vi "Get Event Name.vi"(8 "error in (no error)":errorcluster {"code" format="%.0x"}, 9 "EventNameBufferSize":i32=256 caption="EventNameBufferSize (256)", 10 "EventIndex":i32=1 caption="EventIndex (1)" format="%.0g", 11 "instrument handle":refnum<k15>) -> (0 "error out":errorcluster {"code" format="%.0x"}, 2 "EventName":string, 3 "instrument handle out":refnum<k15>)   [LabVIEW 2009, in "Keysight XSAn.lvlib"]
doc: "This VI returns the physical repeated capability identifier that corresponds to the one-based index that the user specifies. If the value that the user passes for the EventIndex parameter is less than one or greater than the value of the Event Count property, the VI returns an empty string in the EventName parameter and returns an error. For custom event sources added vith the Add Event Source function, this function returns the event source name in the original casing used when Add Event Source was called.\n\nSupported Models: All supported"
uses:
  <instrlib>/Keysight XSAn/Keysight XSAn.lvlib
  AgXSAn.dll
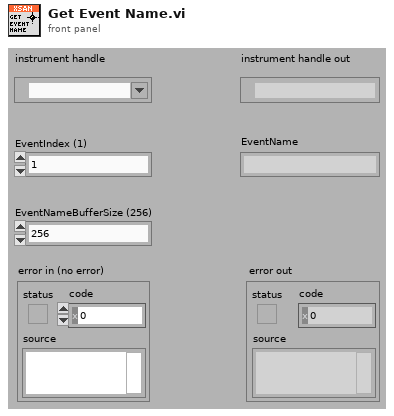
[diagram p1: front panel]
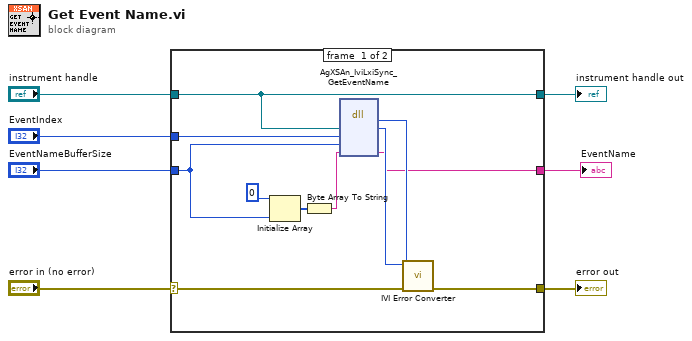
[diagram p0: block diagram]
diagram:
  n1 = case shown="No Error" "error in (no error)" {
    selector: "error in (no error)" -> [w16 w20]
    tunnel: [w15 w20] -> w7
    tunnel: "instrument handle" -> [w9 w19]
    tunnel: "EventIndex" -> [w14 _]
    tunnel: "EventNameBufferSize" -> [w8 _]
    tunnel: [w10 _] -> w2
    tunnel: [w9 w19] -> w1
    frame #0 {
      n2 = Initialize Array(u8 0 ("element"), w8) -> (w12:u8[])
      n3 = Byte Array To String(unsigned byte array=w12) -> (string=w13:string)
      n4 = dll-call lib="AgXSAn**.dll" fn="AgXSAn_IviLxiSync_GetEventName"("Vi"=w9, "EventIndex"=w14, "EventNameBufferSize"=w8, "EventName"=w13) -> (w17:i32, "Vi"=w18:u32, "EventName"=w10:string)  [unwired: 5 in, 2 out]
      n5 = call <instrlib>:"IVI Error Converter.vi"("error in (no error)"=w16, "IVI error code (0)"=w17, "instrument handle"=w18) -> ("error out"=w15:errorcluster)  [unwired: 7 in, 1 out]
    }
    frame #1 {
    }
  }
  "error out" <- w7
  "instrument handle out" <- w1
  "EventName" <- w2
